vi "PlaySequence.vi"(8 "error in (no error)":errorcluster, 10 "Sequence":u8(ring) items=["Last", "Longest"], 11 "Simon_Engine in":refnum<class "Simon_Engine.lvclass">) -> (0 "error out":errorcluster, 3 "Simon_Engine out":refnum<class "Simon_Engine.lvclass">)   [LabVIEW 2019, in "Simon_Engine.lvclass"]
doc: "Plays the sequence of LEDs by blinking them in a certain orded."
uses:
  Simon_Engine.lvclass
  Simon_Engine.lvclass/Simon_Engine.ctl
  LED/LED Class/LED.lvclass/LED.ctl
  LED/LED Class/LED.lvclass
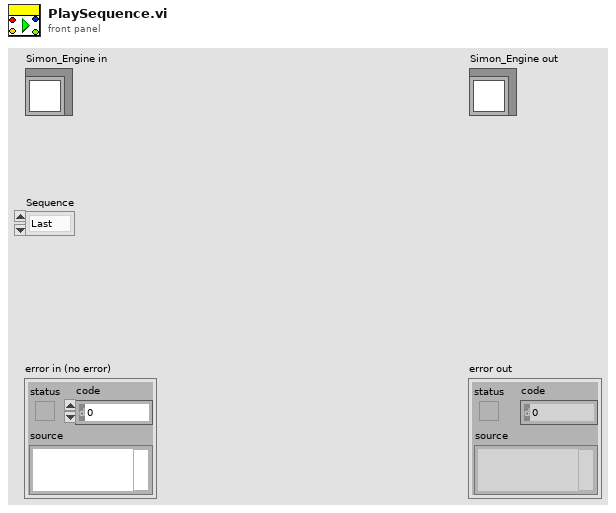
[diagram p1: front panel]
types:
  T1 = enum8{"Enabled", "Disabled", "Disabled and Grayed Out"}
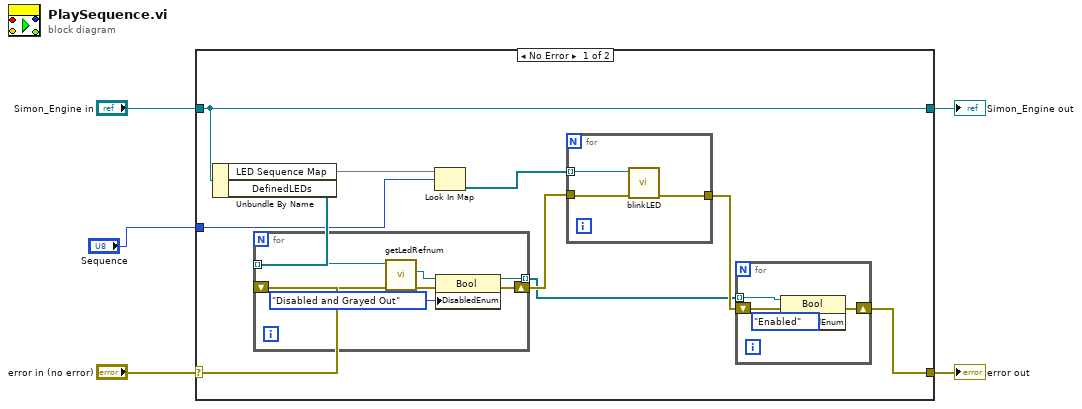
[diagram p0: block diagram]
diagram:
  n1 = case shown="No Error" "error in (no error)" {
    selector: "error in (no error)" -> [w14 w31]
    tunnel: [w11 w31] -> w4
    tunnel: [w15 w30] -> w2
    tunnel: "Simon_Engine in" -> [w15 w30]
    tunnel: "Sequence" -> [w6 _]
    frame No Error {
      n2 = Unbundle By Name(w15) -> ("LED Sequence Map"=w7:map{u8, refnum<class "LED.lvclass">[]}, "DefinedLEDs"=w10:refnum<class "LED.lvclass">[])
      n3 = for {
        shift-right: [w25] -> w12
        shift-left: w14 -> [w26]
        tunnel: w10 -> [w23] mode=indexing
        tunnel: [w21] -> w9 mode=indexing
        n4 = call "getLedRefnum.vi"("error in (no error)"=w26, "LED in"=w23) -> ("error out"=w24:errorcluster, "LED Refnum"=w22:refnum<vi>)  [unwired: 7 in, 1 out]
        n5 = property class="Bool"(reference=w22, error in=w24, "DisabledEnum"=T1."Disabled and Grayed Out" ("Disabled")) -> (reference out=w21:refnum<vi>, error out=w25:errorcluster)
      }
      n6 = Look In Map(map=w7, key=w6) -> (value=w8:refnum<class "LED.lvclass">[])  [unwired: 1 in, 1 out]
      n7 = for {
        tunnel: w8 -> [w29] mode=indexing
        tunnel: w12 -> [w28]
        tunnel: [w27] -> w13
        n8 = call "blinkLED.vi"("error in (no error)"=w28, "LED in"=w29) -> ("error out"=w27:errorcluster)  [unwired: 8 in, 1 out]
      }
      n9 = for {
        shift-right: [w18] -> w11
        shift-left: w13 -> [w19]
        tunnel: w9 -> [w17] mode=indexing
        n10 = property class="Bool"(reference=w17, error in=w19, "DisabledEnum"=T1."Enabled" ("Disabled")) -> (error out=w18:errorcluster)  [unwired: 1 out]
      }
    }
    frame Error {
    }
  }
  "error out" <- w4
  "Simon_Engine out" <- w2
